vi "Cluster Array To Memory Map.vi"(9 "Address Min in":u32 format="%.0x", 10 "Address Max in":u32 format="%.0x", 11 "Array in":T1(array[cluster]) {"CheckSUM" format="%x"}) -> (1 "Address Min out":u32 format="%.0x", 2 "Address Max out":u32 format="%.0x", 3 "Array out":u8[](array[numeric]) format="%.0x")   [LabVIEW 2018]
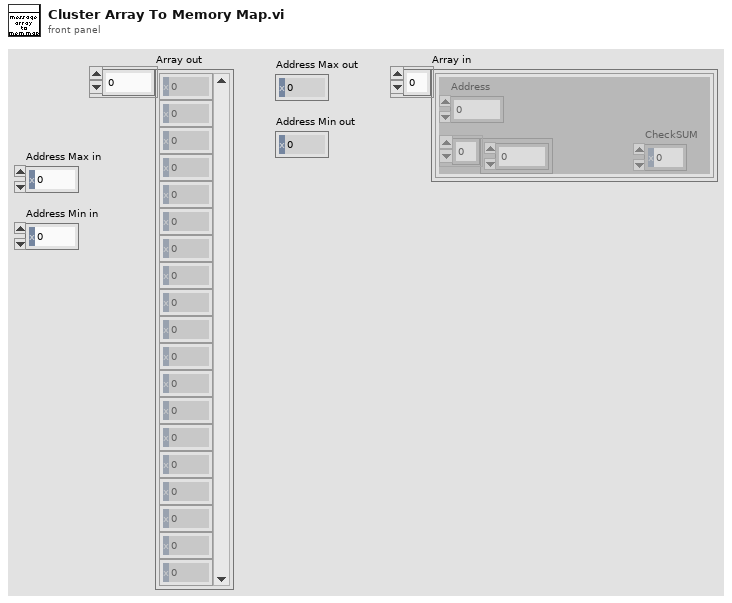
[diagram p1: front panel]
types:
  T1 = cluster{"Address":u32, "Data":u8[], "CheckSUM":u32}[]
  T2 = cluster{"Address":u32, "Data":u8[], "CheckSUM":u32}
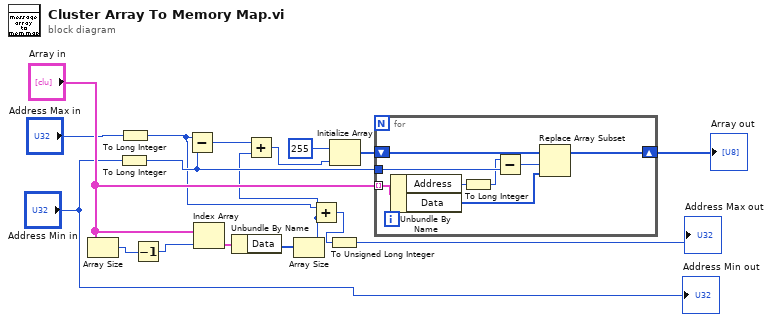
[diagram p0: block diagram]
diagram:
  n1 = Array Size(array="Array in") -> (size(s)=w11:i32)
  n2 = To Long Integer(number="Address Min in") -> (32bit integer=w7:i32)
  n3 = To Long Integer(number="Address Max in") -> (32bit integer=w1:i32)
  n4 = Decrement(x=w11) -> (x-1=w16:i32)
  n5 = Subtract(x=w1, y=w7) -> (x-y=w15:i32)
  n6 = Index Array(array="Array in", index=w16) -> (element=w13:T2)
  n7 = Unbundle By Name(w13) -> ("Data"=w14:u8[])
  n8 = Array Size(array=w14) -> (size(s)=w2:i32)
  n9 = Add(x=w15, y=w2) -> (x+y=w6:i32)
  n10 = Add(x=w1, y=w2) -> (x+y=w4:i32)
  n11 = To Unsigned Long Integer(number=w4) -> (unsigned 32bit integer=→"Address Max out":u32)
  n12 = Initialize Array(u8 255 ("element"), w6) -> (w10:u8[])
  n13 = for {
    tunnel: "Array in" -> [w25] mode=indexing
    tunnel: w7 -> [w23]
    shift-right: [w18] -> w17
    shift-left: w10 -> [w24]
    n14 = Unbundle By Name(w25) -> ("Address"=w22:u32, "Data"=w19:u8[])
    n15 = To Long Integer(number=w22) -> (32bit integer=w21:i32)
    n16 = Subtract(x=w21, y=w23) -> (x-y=w20:i32)
    n17 = Replace Array Subset(array=w24, new element=w19, index=w20) -> (w18:u8[])
  }
  "Array out" <- w17
  "Address Min out" <- "Address Min in"
